vi "Rotation platform.vi"(5 "Revolution (0-0.5)":dbl=0.25 min=0.0 max=0.5 format="%#.2g", 7 "Rotation speed (RPM)":dbl min=0.0 max=50.0 step=0.1 format="%#.2g", 8 "Wait?":bool=TRUE, 9 "Direction":enum16{"Counter clock", "Clock"}(ring), 10 "Pump number":i32=1 min=1 max=9 step=1, 11 "Rotation COM":refnum<visa-resource-name>="COM28") -> ()   [LabVIEW 2017]
uses:
  <instrlib>/Masterflex/Masterflex.lvlib
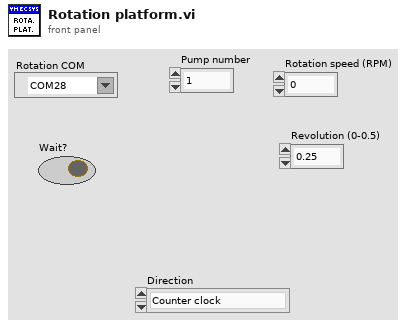
[diagram p1: front panel]
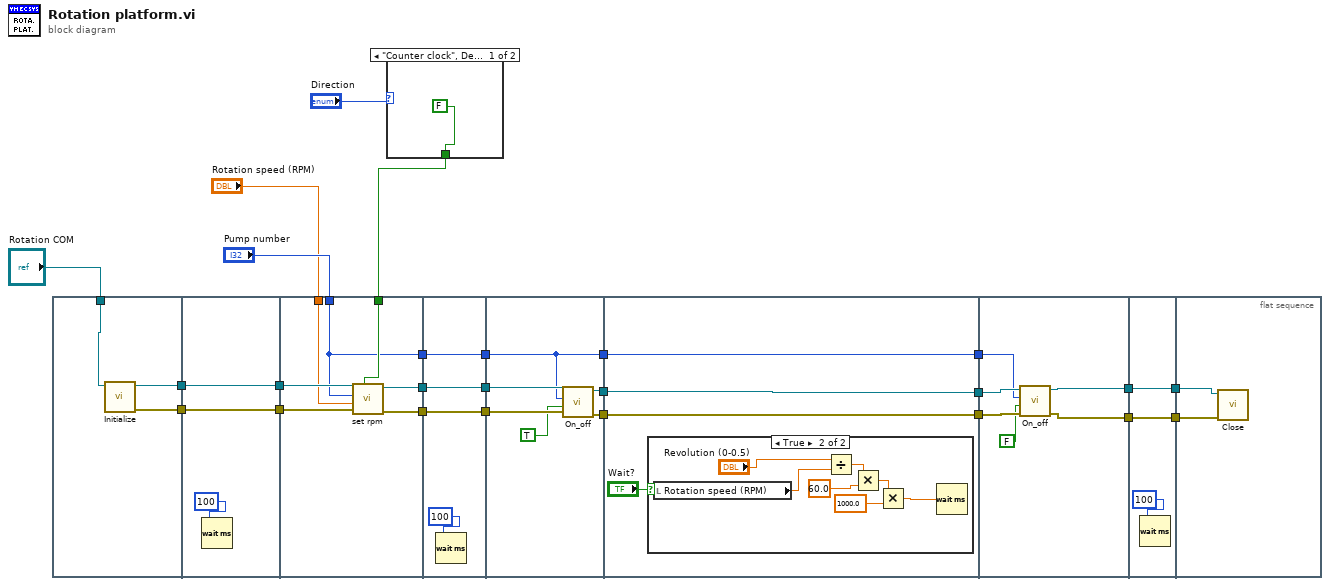
[diagram p0: block diagram]
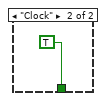
[diagram p2: hidden frame]
diagram:
  n1 = flat-sequence {
    tunnel: "Rotation COM" -> [w28]
    tunnel: [w27] -> w22
    tunnel: [w26] -> w20
    tunnel: [w30] -> w23
    tunnel: w22 -> [w30]
    tunnel: [w29] -> w21
    tunnel: w20 -> [w29]
    tunnel: "Pump number" -> [w32]
    tunnel: w23 -> [w38]
    tunnel: w21 -> [w37]
    tunnel: "Rotation speed (RPM)" -> [w36]
    tunnel: w1 -> [w35]
    tunnel: [w34] -> w17
    tunnel: [w33] -> w15
    tunnel: [w32] -> w13
    tunnel: [w41] -> w18
    tunnel: w17 -> [w41]
    tunnel: [w40] -> w16
    tunnel: w15 -> [w40]
    tunnel: [w39] -> w14
    tunnel: w13 -> [w39]
    tunnel: w18 -> [w48]
    tunnel: w16 -> [w47]
    tunnel: w14 -> [w43]
    tunnel: [w45] -> w11
    tunnel: [w44] -> w9
    tunnel: [w43] -> w7
    tunnel: [w52] -> w12
    tunnel: w11 -> [w52]
    tunnel: [w51] -> w10
    tunnel: w9 -> [w51]
    tunnel: [w50] -> w8
    tunnel: w7 -> [w50]
    tunnel: w12 -> [w65]
    tunnel: w10 -> [w64]
    tunnel: w8 -> [w63]
    tunnel: [w61] -> w5
    tunnel: [w60] -> w3
    tunnel: [w67] -> w6
    tunnel: w5 -> [w67]
    tunnel: [w66] -> w4
    tunnel: w3 -> [w66]
    tunnel: w6 -> [w70]
    tunnel: w4 -> [w69]
    frame #0 {
      n2 = call <instrlib>:"Initialize.vi"("VISA resource name"=w28) -> ("error out"=w26:errorcluster, "VISA resource name out"=w27:refnum<visa-resource-name>)  [unwired: 9 in]
    }
    frame #1 {
      n3 = Wait (ms)(milliseconds to wait=u32 100) -> ()  [unwired: 1 out]
    }
    frame #2 {
      n4 = call <instrlib>:"set rpm.vi"("Clock/counter"=w35, "error in (no error)"=w37, "RPM"=w36, "Pump number"=w32, "VISA resource name"=w38) -> ("error out"=w33:errorcluster, "VISA resource name out"=w34:refnum<visa-resource-name>)  [unwired: 3 in, 2 out]
    }
    frame #3 {
      n5 = Wait (ms)(milliseconds to wait=u32 100) -> ()  [unwired: 1 out]
    }
    frame #4 {
      n6 = call <instrlib>:"On_off.vi"("error in (no error)"=w47, "On/off"=TRUE, "Pump number"=w43, "VISA resource name"=w48) -> ("error out"=w44:errorcluster, "VISA resource name out"=w45:refnum<visa-resource-name>)  [unwired: 5 in, 1 out]
    }
    frame #5 {
      n7 = case shown="True" "Wait?" {
        frame False {
        }
        frame True {
          n8 = local read "Rotation speed (RPM)"() -> (w57:dbl)
          n9 = Divide(x="Revolution (0-0.5)", y=w57) -> (x/y=w59:dbl)
          n10 = Multiply(x=w59, y=60.0) -> (x*y=w55:dbl)
          n11 = Multiply(x=w55, y=1000.0) -> (x*y=w53:dbl)
          n12 = Wait (ms)(milliseconds to wait=w53) -> ()  [unwired: 1 out]
        }
      }
    }
    frame #6 {
      n13 = call <instrlib>:"On_off.vi"("error in (no error)"=w64, "On/off"=FALSE, "Pump number"=w63, "VISA resource name"=w65) -> ("error out"=w60:errorcluster, "VISA resource name out"=w61:refnum<visa-resource-name>)  [unwired: 5 in, 1 out]
    }
    frame #7 {
      n14 = Wait (ms)(milliseconds to wait=u32 100) -> ()  [unwired: 1 out]
    }
    frame #8 {
      n15 = call <instrlib>:"Close.vi"("error in (no error)"=w69, "VISA resource name"=w70) -> ()  [unwired: 9 in, 1 out]
    }
  }
  n16 = case shown="\"Counter clock\", Default" "Direction" {
    tunnel: [FALSE TRUE] -> w1
    frame "Counter clock", Default {
    }
    frame "Clock" {
    }
  }
